vi "Undo.vi"(8 "error in (no error)":errorcluster, 11 "Map Model in":refnum<class "Map Model.lvclass">) -> (0 "error out":errorcluster, 3 "Map Model out":refnum<class "Map Model.lvclass">)   [LabVIEW 2020, in "Map Model.lvlib" / "Map Model.lvclass"]
uses:
  Map Model.lvclass
  Map Model.lvclass/Map Model.ctl
  Tools/Undoable Tool/Undoable Tool.lvclass/Undoable Tool.ctl
  Tools/Undoable Tool/Undoable Tool.lvclass
  Stack/Stack.lvclass
panel:
  # "NOTICE -- YOU MUST LEAVE THIS NOTICE IN PLACE.\n\nCopyright (c) 2017, LIANG LIU Shawn.Liu.cn@gmail.com\nAll rights reserved.\n\nRedistribution and use in source and binary forms, with or without modification, are permitted provided that the following conditions are met:\n-Redistributions of source code must retain the above copyright notice, this list of conditions and the following disclaimer.\n-Redistributions in binary form must reproduce the above copyright notice, this list of conditions and the following disclaimer in the documentation and/or other materials provided with the distribution.\n-Neither the name of the eLp nor the names of its contributors may be used to endorse or promote products derived from this software without specific prior written permission.\n\nTHIS SOFTWARE IS PROVIDED BY THE COPYRIGHT HOLDERS AND CONTRIBUTORS \"AS IS\" AND ANY EXPRESS OR IMPLIED WARRANTIES, INCLUDING, BUT NOT LIMITED TO, THE IMPLIED WARRANTIES OF MERCHANTABILITY AND FITNESS FOR A PARTICULAR PURPOSE ARE DISCLAIMED. IN NO EVENT SHALL THE COPYRIGHT HOLDER OR CONTRIBUTORS BE LIABLE FOR ANY DIRECT, INDIRECT, INCIDENTAL, SPECIAL, EXEMPLARY, OR CONSEQUENTIAL DAMAGES (INCLUDING, BUT NOT LIMITED TO, PROCUREMENT OF SUBSTITUTE GOODS OR SERVICES; LOSS OF USE, DATA, OR PROFITS; OR BUSINESS INTERRUPTION) HOWEVER CAUSED AND ON ANY THEORY OF LIABILITY, WHETHER IN CONTRACT, STRICT LIABILITY, OR TORT (INCLUDING NEGLIGENCE OR OTHERWISE) ARISING IN ANY WAY OUT OF THE USE OF THIS SOFTWARE, EVEN IF ADVISED OF THE POSSIBILITY OF SUCH DAMAGE."
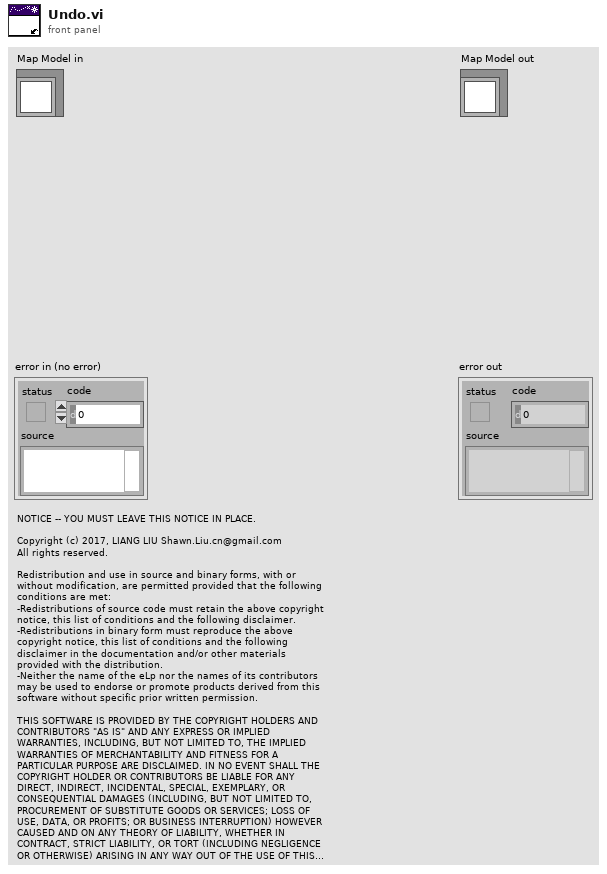
[diagram p1: front panel]
types:
  T1 = enum8{"Enabled", "Disabled", "Disabled and Grayed Out"}
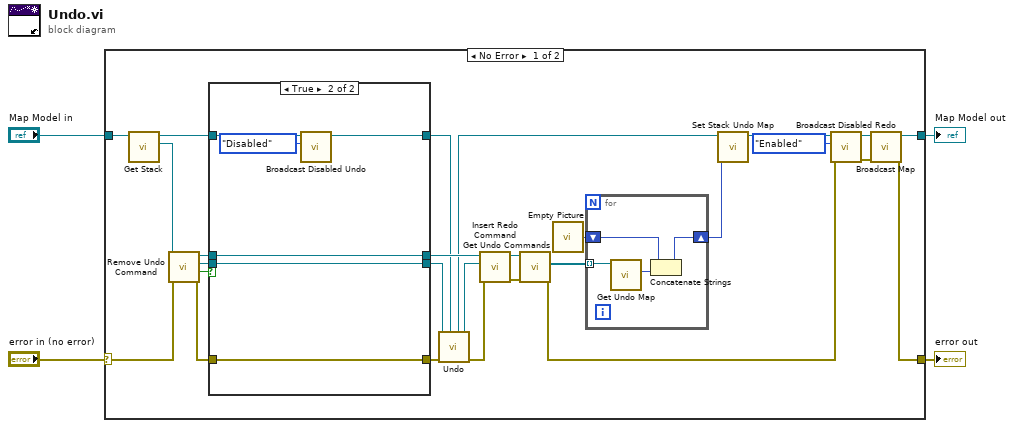
[diagram p0: block diagram]
diagram:
  n1 = case shown="No Error" "error in (no error)" {
    selector: "error in (no error)" -> [w28 w47]
    tunnel: "Map Model in" -> [w31 w46]
    tunnel: [w30 w46] -> w3
    tunnel: [w29 w47] -> w2
    frame No Error {
      n2 = call "Get Stack.vi"("Map Model in"=w31) -> ("Stack"=w27:refnum<class "Stack.lvclass">, "Map Model out"=w23:refnum<class "Map Model.lvclass">)  [unwired: 9 in]
      n3 = call "Remove Undo Command.vi"("error in (no error)"=w28, "Stack in"=w27) -> ("error out"=w13:errorcluster, "Empty"=w26:bool, "Undo Command"=w24:refnum<class "Undoable Tool.lvclass">, "Stack out"=w25:refnum<class "Stack.lvclass">)  [unwired: 6 in]
      n4 = case shown="True" w26 {
        tunnel: w25 -> [w39 w44]
        tunnel: w24 -> [w38 w45]
        tunnel: [w38 w45] -> w17
        tunnel: [w39 w44] -> w22
        tunnel: w23 -> [w37 w43]
        tunnel: [w37 w41] -> w15
        tunnel: w13 -> [w36 w42]
        tunnel: [w36 w42] -> w12
        frame False {
        }
        frame True {
          n5 = call "Broadcast Disabled Undo.vi"("Disabled Undo"=T1."Disabled", "Map Model in"=w43) -> ("Map Model out"=w41:refnum<class "Map Model.lvclass">)  [unwired: 8 in, 1 out]
        }
      }
      n6 = call-dynamic "Undo.vi"("Map Model in"=w15, "error in (no error)"=w12, "Undoable Tool in"=w17) -> ("error out"=w10:errorcluster, "Undoable Tool out"=w16:refnum<class "Undoable Tool.lvclass">, "Map Model out"=w14:refnum<class "Map Model.lvclass">)  [unwired: 6 in]
      n7 = call "Insert Redo Command.vi"("error in (no error)"=w10, "Redo Command"=w16, "Stack in"=w22) -> ("error out"=w20:errorcluster, "Stack out"=w21:refnum<class "Stack.lvclass">)  [unwired: 5 in, 2 out]
      n8 = call "Get Undo Commands.vi"("error in (no error)"=w20, "Stack in"=w21) -> ("error out"=w6:errorcluster, "Undo Commands"=w19:refnum<class "Undoable Tool.lvclass">[])  [unwired: 7 in, 1 out]
      n9 = call "Empty Picture"() -> ("empty picture"=w18:picture)
      n10 = for {
        tunnel: w19 -> [w35] mode=indexing
        shift-right: [w32] -> w11
        shift-left: w18 -> [w33]
        n11 = call "Get Undo Map.vi"("Undoable Tool in"=w35) -> ("Undo Map"=w34:picture)  [unwired: 9 in, 1 out]
        n12 = Concatenate Strings(w33, w34) -> (w32:picture)
      }
      n13 = call "Set Stack Undo Map.vi"("Stack Undo Map"=w11, "Map Model in"=w14) -> ("Map Model out"=w9:refnum<class "Map Model.lvclass">)  [unwired: 9 in]
      n14 = call "Broadcast Disabled Redo.vi"("error in (no error)"=w6, "Disabled Redo"=T1."Enabled", "Map Model in"=w9) -> ("error out"=w5:errorcluster, "Map Model out"=w8:refnum<class "Map Model.lvclass">)  [unwired: 7 in]
      n15 = call "Broadcast Map.vi"("error in (no error)"=w5, "Map Model in"=w8) -> ("error out"=w29:errorcluster, "Map Model out"=w30:refnum<class "Map Model.lvclass">)  [unwired: 8 in]
    }
    frame Error {
    }
  }
  "error out" <- w2
  "Map Model out" <- w3
